vi "Init Select Module Ring.vi"(8 "error in (no error)":errorcluster, 11 "Select Module MCL Ref":refnum<vi>) -> (0 "error out":errorcluster, 1 "Module MCL Value":i32=-1, 3 "Value for All Modules":i32)   [LabVIEW 2014, in "Configurable.lvlib"]
doc: "Initialize the strings and values in the module selector ring.\n_____\nBased on Delacor QMH Project Template 4.0.0.47."
uses:
  Configurable.lvlib
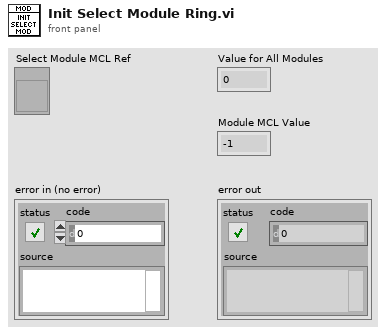
[diagram p1: front panel]
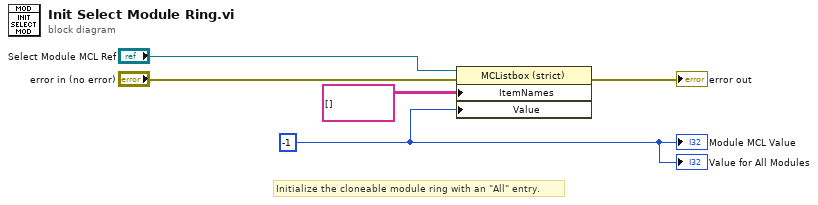
[diagram p0: block diagram]
diagram:
  w1 = -1 ("element")
  # "Initialize the cloneable module ring with an \"All\" entry."
  n1 = property on="Property Node" class="MCListbox (strict)"(reference="Select Module MCL Ref", error in="error in (no error)", "ItemNames"=string[][] [] ("Item Names"), "Value"=w1) -> (error out=→"error out":errorcluster)  [unwired: 1 out]
  "Value for All Modules" <- w1
  "Module MCL Value" <- w1
